vi "Teleop.vi"(10 "Match Info":T1={"Autonomous Elapsed Seconds"=0.0, "TeleOp Elapsed Seconds"=0.0, "Disabled Elapsed Seconds"=0.0, "Visited Autonomous"=FALSE, "Visited TeleOp"=FALSE, "Visited Disabled"=FALSE, "Autonomous Settings"={"Autonomous Style"=enum."Independent", "VI Refnum"=refnum}}, 11 "Call Context":T2) -> ()   [LabVIEW 2012]
doc: "This VI is called for each TeleOp packet received from the DS where the robot is not disabled. It is often used to read from the joysticks and update I/O or to update setpoints for timed control loops. It should complete and return within 20 milliseconds or it may miss DS packets."
uses:
  <vilib>/Rock Robotics/WPI/DriverStation/WPI_DriverStationDerivedRobotMode.ctl
  <vilib>/Rock Robotics/WPI/DriverStation/WPI_DriverStationMatch Info.ctl
  Robot Global Data.vi
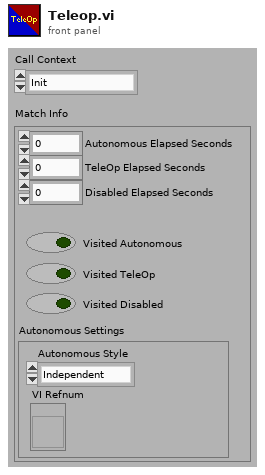
[diagram p1: front panel]
types:
  T1 = typedef "WPI_DriverStationMatch Info.ctl" = cluster{"Autonomous Elapsed Seconds":dbl, "TeleOp Elapsed Seconds":dbl, "Disabled Elapsed Seconds":dbl, "Visited Autonomous":bool, "Visited TeleOp":bool, "Visited Disabled":bool, "Autonomous Settings":cluster{"Autonomous Style":enum16{"Iterative", "Independent"}, "VI Refnum":refnum<vi>}}
  T2 = typedef "WPI_DriverStationDerivedRobotMode.ctl" = enum16{"Init", "Execute", "Stop"}
  T3 = typedef "WPI_JoystickButtonState.ctl" = cluster{"Button 1":bool, "Button 2":bool, "Button 3":bool, "Button 4":bool, "Button 5":bool, "Button 6":bool, "Button 7":bool, "Button 8":bool, "Button 9":bool, "Button 10":bool, "Button 11":bool, "Button 12":bool}
  T4 = cluster{"axis 1 (x)":dbl, "axis 2 (y)":dbl, "axis 3 (throttle)":dbl, "axis 4":dbl, "axis 5":dbl, "axis 6":dbl}
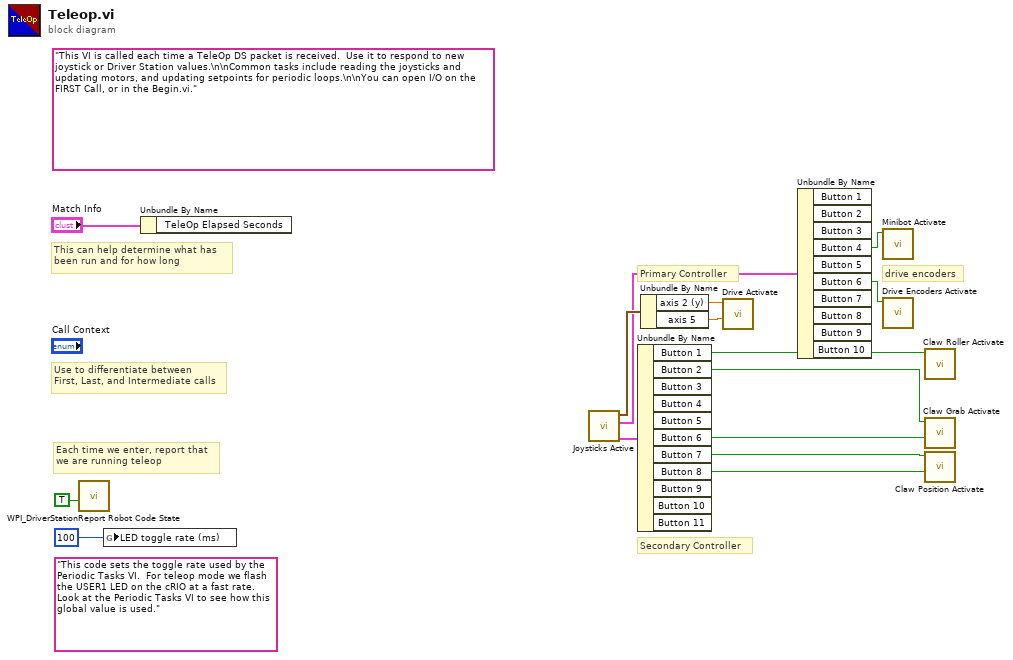
[diagram p0: block diagram]
diagram:
  (unwired) "This code sets the toggle rate used by the Periodic Tasks VI.  For teleop mode we flash the USER1 LED on the cRIO at a fast rate.  Look at the Periodic Tasks VI to see how this global value is used."
  (unwired) "This VI is called each time a TeleOp DS packet is received.  Use it to respond to new joystick or Driver Station values.\n\nCommon tasks include reading the joysticks and updating motors, and updating setpoints for periodic loops.\n\nYou can open I/O on the FIRST Call, or in the Begin.vi."
  # "drive encoders"
  # "Secondary Controller"
  # "Primary Controller"
  # "Each time we enter, report that\nwe are running teleop"
  # "Use to differentiate between\nFirst, Last, and Intermediate calls"
  # "This can help determine what has\nbeen run and for how long"
  n1 = call <vilib>:"WPI_DriverStationReport Robot Code State.vi"("TeleOp"=TRUE ("Autonomous")) -> ()  [unwired: 10 in, 1 out]
  n2 = global write "Robot Global Data.vi" "LED toggle rate (ms)"(u32 100 ("LED ms toggle rate")) -> ()
  n3 = Unbundle By Name("Match Info") -> ()  [unwired: 1 out]
  n4 = call "Joysticks Active.vi"() -> ("Secondary Controller Buttons"=w10:T3, "Primary Controller Buttons"=w11:T3, "Primary Controller Axes"=w12:T4)  [unwired: 8 in, 1 out]
  n5 = Unbundle By Name(w10) -> ("Button 1"=w6:bool, "Button 2"=w5:bool, "Button 6"=w4:bool, "Button 7"=w3:bool, "Button 8"=w2:bool)  [unwired: 6 out]
  n6 = Unbundle By Name(w12) -> ("axis 2 (y)"=w9:dbl, "axis 5"=w8:dbl)
  n7 = call "Drive Activate.vi"("Right Joystick"=w8, "Left Joystick"=w9) -> ()  [unwired: 10 in]
  n8 = Unbundle By Name(w11) -> ("Button 4"=w1:bool, "Button 6"=w7:bool)  [unwired: 8 out]
  n9 = call "Minibot Activate.vi"("Fire Minibot"=w1) -> ()  [unwired: 11 in]
  n10 = call "Drive Encoders Activate.vi"("Encoder Reset"=w7) -> ()  [unwired: 10 in, 1 out]
  n11 = call "Claw Roller Activate.vi"("Start Rollers"=w6) -> ()  [unwired: 11 in]
  n12 = call "Claw Grab Activate.vi"("Let Go"=w4, "Grab"=w5) -> ()  [unwired: 10 in]
  n13 = call "Claw Position Activate.vi"("Claw Retract"=w2, "Claw Extend"=w3) -> ()  [unwired: 10 in]
